vi "FireUserEvent_1.vi"(2 "error in (no error)":errorcluster, 3 "UserEvent":T1, 4 "Enum":enum16{"GetRef", "Fire", "Release"}(ring)) -> (0 "error out":errorcluster, 1 "UserEvent 2":refnum<user-event>)   [LabVIEW 2011]
uses:
  UserEvent.ctl
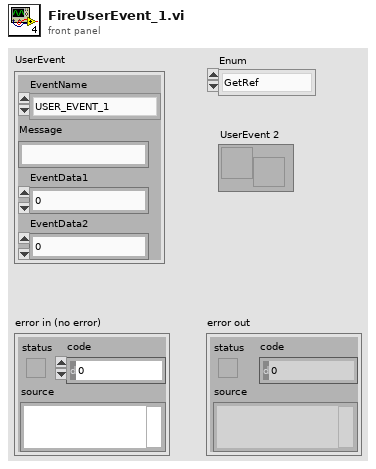
[diagram p1: front panel]
types:
  T1 = typedef "UserEvent.ctl" = cluster{"EventName":enum16{"USER_EVENT_1", "USER_EVENT_2", "USER_EVENT_3", "USER_EVENT_4", "USER_EVENT_5", "USER_EVENT_6", "USER_EVENT_7", "USER_EVENT_8", "USER_EVENT_9", "USER_EVENT_10"}, "Message":string, "EventData1":dbl, "EventData2":dbl}
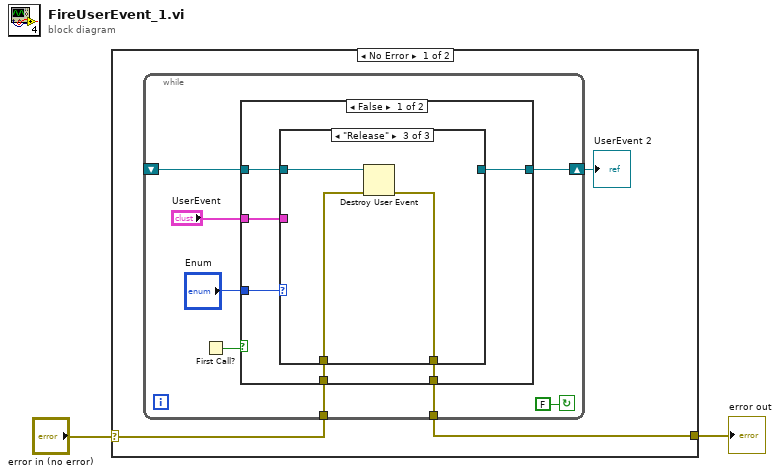
[diagram p0: block diagram]
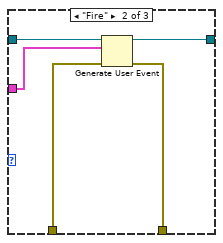
[diagram p3: hidden frame]
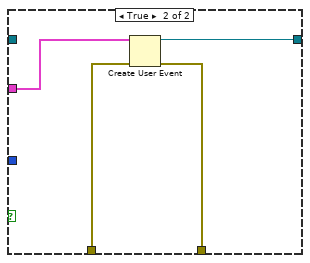
[diagram p4: hidden frame]
diagram:
  n1 = case shown="No Error" "error in (no error)" {
    selector: "error in (no error)" -> [w5 w34]
    tunnel: [w3 w34] -> w1
    frame No Error {
      n2 = while {
        shift-right: [w9] -> w4
        shift-left: _ -> [w8]
        tunnel: w5 -> [w7]
        tunnel: [w6] -> w3
        stop <- FALSE continue-if-true
        n3 = First Call?() -> (First Call?: T/F=w13:bool)
        n4 = case shown="False" w13 {
          tunnel: "Enum" -> [w19 _]
          tunnel: "UserEvent" -> [w18 w33]
          tunnel: [w16 w32] -> w9
          tunnel: w8 -> [w17 _]
          tunnel: w7 -> [w15 w31]
          tunnel: [w14 w30] -> w6
          frame False {
            n5 = case shown="\"Release\"" w19 {
              tunnel: w18 -> [_ w24 _]
              tunnel: w17 -> [w21 w26 w29]
              tunnel: [w21 w25 _] -> w16
              tunnel: w15 -> [w20 w23 w28]
              tunnel: [w20 w22 w27] -> w14
              frame "GetRef", Default {
              }
              frame "Fire" {
                n6 = Generate User Event(user event=w26, event data cluster=w24, error in=w23) -> (user event out=w25:refnum<user-event>, error out=w22:errorcluster)
              }
              frame "Release" {
                n7 = Destroy User Event(user event=w29, error in=w28) -> (error out=w27:errorcluster)
              }
            }
          }
          frame True {
            n8 = Create User Event(user event datatype=w33, error in=w31) -> (user event=w32:refnum<user-event>, error out=w30:errorcluster)
          }
        }
      }
      "UserEvent 2" <- w4
    }
    frame Error {
    }
  }
  "error out" <- w1
